vi "习题3.6.vi"() -> ()   [LabVIEW 2018]
panel:
  in  "数字":dbl
  out "布尔":bool
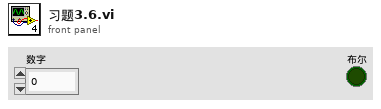
[diagram p1: front panel]
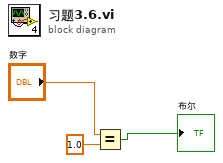
[diagram p0: block diagram]
diagram:
  n1 = Equal?(x="数字", y=1.0) -> (x = y?=→"布尔":bool)
